vi "niRFSG Get Session Reference.vi"(0 "instrument handle":refnum<k15>, 11 "error in":errorcluster {"code" format="%.0x"}) -> (4 "instrument handle out":refnum<k15>, 6 "session reference":refnum<k20>, 15 "error out":errorcluster {"code" format="%.0x"})   [LabVIEW 2014]
doc: "Extracts a session that can be passed to NI-TClk VIs. Session References are of generic data type, which means that the corresponding wires are blue-green, unlike the wires for regular instrument driver sessions.\n\n<B>Supported Devices</B>: NI 5673/5673E, NI 5840"
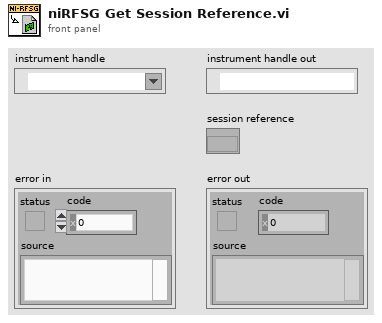
[diagram p1: front panel]
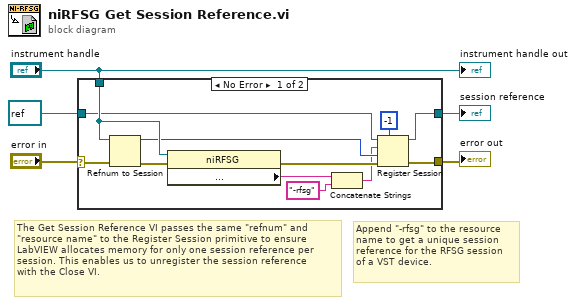
[diagram p0: block diagram]
diagram:
  # "Append \"-rfsg\" to the resource\nname to get a unique session\nreference for the RFSG session\nof a VST device."
  # "The Get Session Reference VI passes the same \"refnum\" and \n\"resource name\" to the Register Session primitive to ensure \nLabVIEW allocates memory for only one session reference per\nsession. This enables us to unregister the session reference \nwith the Close VI."
  n1 = case shown="No Error" "error in" {
    selector: "error in" -> [w15 w19]
    tunnel: [w16 w19] -> w2
    tunnel: "instrument handle" -> [w13 _]
    tunnel: [w17 w18] -> w4
    tunnel: refnum<k20> refnum ("session reference") -> [w9 w18]
    frame No Error {
      n2 = Refnum to Session(4:w15, 7:w13) -> (0:w14:errorcluster, 3:w10:u64)
      n3 = property class="niRFSG"(reference=w13, error in=w14) -> (error out=w12:errorcluster, "Instrument:Inherent IVI Attributes:Advanced Session Information:Resource Descriptor"=w8:string)  [unwired: 1 out]
      n4 = Concatenate Strings(w8, "-rfsg" ("string")) -> (w7:string)
      n5 = Register Session(7:-1 ("cleanup mode (default to class = 0)"), 8:w12, 9:w10, 10:w7, 11:w9) -> (0:w16:errorcluster, 3:w17:refnum<k20>)
    }
    frame Error {
    }
  }
  "session reference" <- w4
  "error out" <- w2
  "instrument handle out" <- "instrument handle"
